vi "find greper points.vi"(2 "Circles":cluster{"x":dbl, "y":dbl, "r":dbl}[](array[cluster]), 3 "Type  2":enum16{"Z", "I", "O", "S", "L", "J", "T", "N"}(ring)=enum."O") -> (0 "gripper":T1, 1 "Type":enum16{"Z", "I", "O", "S", "L", "J", "T", "N"}(ring)=enum."O")   [LabVIEW 2018]
panel:
  out "output variable":i32
  out "dj":dbl[](array[numeric])
  out "di":dbl[](array[numeric])
  out "p2":dbl[](array[numeric])
  out "p1":dbl[](array[numeric])
  out "ok":i32
  out "i":i32
  out "points":cluster{"p1":dbl[], "p2":dbl[]}[](array[cluster])
  out "x":dbl[](array[numeric])
  out "y":dbl[](array[numeric])
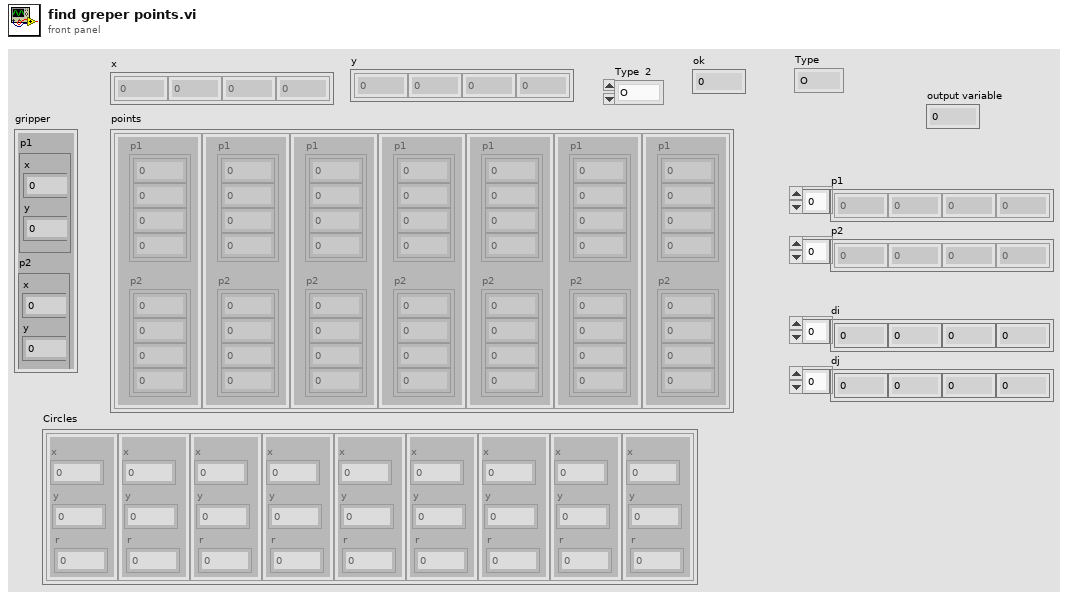
[diagram p1: front panel]
types:
  T1 = cluster{"p1":cluster{"x":dbl, "y":dbl}, "p2":cluster{"x":dbl, "y":dbl}}
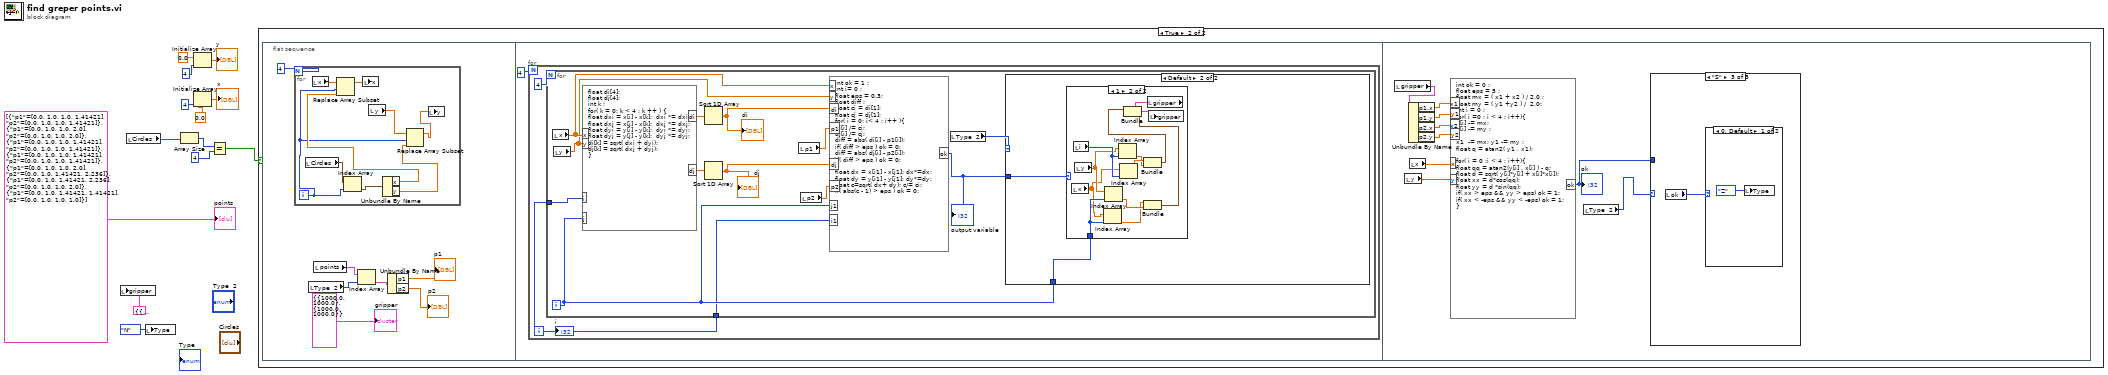
[diagram p0: block diagram]
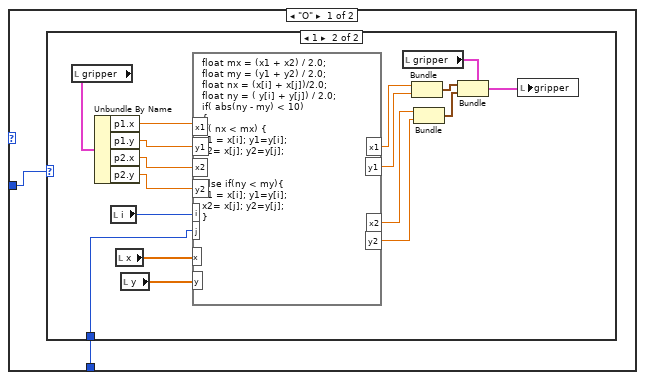
[diagram p3: hidden frame]
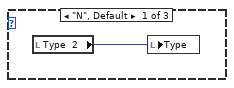
[diagram p6: hidden frame]
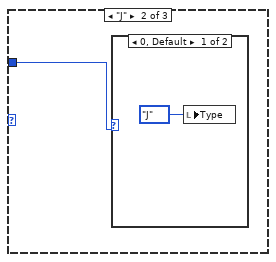
[diagram p7: hidden frame]
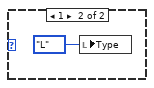
[diagram p8: hidden frame]
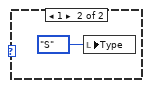
[diagram p9: hidden frame]
diagram:
  n1 = local write "gripper"(T1 {"p1"={"x"=0.0, "y"=0.0}, "p2"={"x"=0.0, "y"=0.0}} ("gripper")) -> ()
  n2 = local read "Circles"() -> (w13:cluster{"x":dbl, "y":dbl, "r":dbl}[])
  n3 = local write "Type"(enum16{"Z", "I", "O", "S", "L", "J", "T", "N"}."N" ("Type")) -> ()
  n4 = Array Size(array=w13) -> (size(s)=w12:i32)
  n5 = Initialize Array(0.0 ("element"), 4 ("dimension size")) -> (→"y":dbl[])
  n6 = Initialize Array(0.0 ("element"), 4 ("dimension size")) -> (→"x":dbl[])
  n7 = Equal?(x=w12, y=4) -> (x = y?=w10:bool)
  n8 = case shown="True" w10 {
    frame False {
    }
    frame True {
      n9 = flat-sequence {
        frame #0 {
          n10 = for {
            N: 4 -> [_]
            i -> [w23]
            n11 = local read "Circles"() -> (w29:cluster{"x":dbl, "y":dbl, "r":dbl}[])
            n12 = local read "x"() -> (w27:dbl[])
            n13 = Index Array(array=w29, index=w23) -> (element=w28:cluster{"x":dbl, "y":dbl, "r":dbl})
            n14 = local read "y"() -> (w24:dbl[])
            n15 = Unbundle By Name(w28) -> ("x"=w26:dbl, "y"=w22:dbl)
            n16 = Replace Array Subset(array=w27, new element=w26, index=w23) -> (w25:dbl[])
            n17 = local write "x"(w25) -> ()
            n18 = Replace Array Subset(array=w24, new element=w22, index=w23) -> (w21:dbl[])
            n19 = local write "y"(w21) -> ()
          }
          n20 = local read "Type  2"() -> (w18:enum16{"Z", "I", "O", "S", "L", "J", "T", "N"})
          n21 = local read "points"() -> (w19:cluster{"p1":dbl[], "p2":dbl[]}[])
          n22 = Index Array(array=w19, index=w18) -> (element=w17:cluster{"p1":dbl[], "p2":dbl[]})
          n23 = Unbundle By Name(w17) -> ("p1"=→"p1":dbl[], "p2"=→"p2":dbl[])
          "gripper" <- T1 {"p1"={"x"=1000.0, "y"=1000.0}, "p2"={"x"=1000.0, "y"=1000.0}} ("gripper")
        }
        frame #1 {
          n24 = for {
            N: 4 -> [_]
            i -> [w31]
            n25 = for {
              N: 4 -> [_]
              tunnel: w31 -> [w45]
              tunnel: w31 -> [w36]
              i -> [w37]
              n26 = local read "x"() -> (w35:dbl[])
              n27 = local read "y"() -> (w34:dbl[])
              n28 = formula code="float di[4];\nfloat dj[4];\nint k ;\nfor( k = 0; k < 4 ; k ++ ) {\nfloat dxi = x[i] - x[k];  dxi *= dxi;\nfloat dxj = x[j] - x[k];  dxj *= dxj;\nfloat dyi = y[i] - y[k];  dyi *= dyi;\nfloat dyj = y[j] - y[k];  dyj *= dyj;\ndi[k] = sqrt( dxi + dyi);\ndj[k] = sqrt( dxj + dyj);\n}"("i"=w45, "j"=w37, "x"=w35, "y"=w34) -> ("di"=w44:dbl[], "dj"=w43:dbl[])
              n29 = Sort 1D Array(array=w44) -> (sorted array=w42:dbl[])
              "di" <- w42
              n30 = Sort 1D Array(array=w43) -> (sorted array=w41:dbl[])
              "dj" <- w41
              n31 = local read "p1"() -> (w39:dbl[])
              n32 = local read "p2"() -> (w40:dbl[])
              n33 = formula code="int ok = 1 ;\nint i= 0 ;\nfloat eps = 0.3;\nfloat diff ;\nfloat ci = di[1];\nfloat cj = dj[1];\nfor( i = 0; i< 4 ; i++ ){\ndi[i] /= ci;\ndj[i] /= cj;\ndiff = abs( di[i] - p1[i]);\nif( diff > eps ) ok = 0;\ndiff = abs( dj[i] - p2[i]);\nif( diff > eps ) ok = 0;\n}\nfloat dx = x[i1] - x[j1]; dx*=dx;\nfloat dy = y[i1] - y[j1]; dy*=dy;\nfloat c=sqrt( dx+ dy); c/= ci;\nif( abs(c - 1) > eps ) ok = 0;"("di"=w42, "dj"=w41, "p1"=w39, "p2"=w40, "i1"=w36, "j1"=w37, "x"=w35, "y"=w34) -> ("ok"=w38:i32)
              "output variable" <- w38
              n34 = local read "Type  2"() -> (w33:enum16{"Z", "I", "O", "S", "L", "J", "T", "N"})
              n35 = case shown="Default" w33 {
                tunnel: w38 -> [w46 w66]
                tunnel: w37 -> [w47 w65]
                frame "O" {
                  n36 = case shown="1" w46 {
                    tunnel: w47 -> [_ w50]
                    frame 0, Default {
                    }
                    frame 1 {
                      n37 = local read "gripper"() -> (w60:T1)
                      n38 = Unbundle By Name(w60) -> ("p1.x"=w55:dbl, "p1.y"=w54:dbl, "p2.x"=w53:dbl, "p2.y"=w52:dbl)
                      n39 = local read "i"() -> (w51:i32)
                      n40 = local read "x"() -> (w49:dbl[])
                      n41 = local read "y"() -> (w48:dbl[])
                      n42 = formula code="float mx = (x1 + x2) / 2.0;\nfloat my = (y1 + y2) / 2.0;\nfloat nx = (x[i] + x[j])/2.0;\nfloat ny = ( y[i] + y[j]) / 2.0;\nif( abs(ny - my) < 10)\n{\nif( nx < mx) {\nx1 = x[i]; y1=y[i];\nx2= x[j]; y2=y[j];\n}\n}\nelse if(ny < my){\nx1 = x[i]; y1=y[i];\nx2= x[j]; y2=y[j];\n}"("x1"=w55, "y1"=w54, "x2"=w53, "y2"=w52, "i"=w51, "j"=w50, "x"=w49, "y"=w48) -> ("x1"=w59:dbl, "y1"=w58:dbl, "x2"=w57:dbl, "y2"=w56:dbl)
                      n43 = local read "gripper"() -> (w64:T1)
                      n44 = Bundle("x1"=w59, "y1"=w58) -> (w62:cluster{"x1":dbl, "y1":dbl})  [unwired: 1 in]
                      n45 = Bundle("x2"=w57, "y2"=w56) -> (w61:cluster{"x2":dbl, "y2":dbl})  [unwired: 1 in]
                      n46 = Bundle(cluster=w64, "p1"=w62, "p2"=w61) -> (w63:T1)
                      n47 = local write "gripper"(w63) -> ()
                    }
                  }
                }
                frame Default {
                  n48 = case shown="1" w66 {
                    tunnel: w65 -> [_ w76]
                    frame 0, Default {
                    }
                    frame 1 {
                      n49 = local read "x"() -> (w70:dbl[])
                      n50 = local read "i"() -> (w72:i32)
                      n51 = local read "y"() -> (w71:dbl[])
                      n52 = Index Array(array=w70, index=w76) -> (element=w73:dbl)
                      n53 = Index Array(array=w71, index=w76) -> (element=w74:dbl)
                      n54 = Index Array(array=w71, index=w72) -> (element=w68:dbl)
                      n55 = Index Array(array=w70, index=w72) -> (element=w69:dbl)
                      n56 = Bundle("element"=w69, "element"=w68) -> (w67:cluster{"element":dbl, "element":dbl})  [unwired: 1 in]
                      n57 = Bundle("element"=w73, "element"=w74) -> (w75:cluster{"element":dbl, "element":dbl})  [unwired: 1 in]
                      n58 = local read "gripper"() -> (w78:T1)
                      n59 = Bundle(cluster=w78, "p1"=w67, "p2"=w75) -> (w77:T1)
                      n60 = local write "gripper"(w77) -> ()
                    }
                  }
                }
              }
            }
            "i" <- w31
          }
        }
        frame #2 {
          n61 = local read "gripper"() -> (w87:T1)
          n62 = local read "y"() -> (w81:dbl[])
          n63 = Unbundle By Name(w87) -> ("p1.x"=w86:dbl, "p1.y"=w85:dbl, "p2.x"=w84:dbl, "p2.y"=w83:dbl)
          n64 = local read "x"() -> (w82:dbl[])
          n65 = formula code="int ok = 0 ;\nfloat eps = 5 ;\nfloat mx = ( x1 + x2 ) / 2.0 ;\nfloat my = ( y1 +y2 ) /  2.0;\nint i = 0 ;\nfor( i =0 ; i < 4 ; i++){\nx[i] -= mx;\ny[i] -= my ;\n}\nx1  -= mx; y1 -= my ;\nfloat q = atan2( y1 , x1);\n\nfor( i = 0 ;i < 4 ; i++){\nfloat qq = atan2(y[i] , x[i] ) - q;\nfloat d = sqrt( y[i]*y[i] + x[i]*x[i]);\nfloat xx = d*cos(qq);\nfloat yy = d *sin(qq);\nif( xx > eps && yy > eps) ok = 1;\nif( xx < -eps && yy < -eps) ok = 1;\n}"("x1"=w86, "y1"=w85, "x2"=w84, "y2"=w83, "x"=w82, "y"=w81) -> ("ok"=w79:i32)
          "ok" <- w79
          n66 = local read "Type  2"() -> (w80:enum16{"Z", "I", "O", "S", "L", "J", "T", "N"})
          n67 = case shown="\"S\"" w80 {
            tunnel: w79 -> [_ w89 _]
            frame "N", Default {
              n68 = local read "Type  2"() -> (w88:enum16{"Z", "I", "O", "S", "L", "J", "T", "N"})
              n69 = local write "Type"(w88) -> ()
            }
            frame "J" {
              n70 = case shown="0, Default" w89 {
                frame 0, Default {
                  n71 = local write "Type"(enum16{"Z", "I", "O", "S", "L", "J", "T", "N"}."J" ("Type  3")) -> ()
                }
                frame 1 {
                  n72 = local write "Type"(enum16{"Z", "I", "O", "S", "L", "J", "T", "N"}."L" ("Type  3")) -> ()
                }
              }
            }
            frame "S" {
              n73 = local read "ok"() -> (w92:i32)
              n74 = case shown="0, Default" w92 {
                frame 0, Default {
                  n75 = local write "Type"(enum16{"Z", "I", "O", "S", "L", "J", "T", "N"}."Z" ("Type  3")) -> ()
                }
                frame 1 {
                  n76 = local write "Type"(enum16{"Z", "I", "O", "S", "L", "J", "T", "N"}."S" ("Type  3")) -> ()
                }
              }
            }
          }
        }
      }
    }
  }
  "points" <- cluster{"p1":dbl[], "p2":dbl[]}[] [{"p1"=[0.0, 1.0, 1.0, 1.41421], "p2"=[0.0, 1.0, 1.0, 1.41421]}, {"p1"=[0.0, 1.0, 1.0, 2.0], "p2"=[0.0, 1.0, 1.0, 2.0]}, {"p1"=[0.0, 1.0, 1.0, 1.41421], "p2"=[0.0, 1.0, 1.0, 1.41421]}, {"p1"=[0.0, 1.0, 1.0, 1.41421], "p2"=[0.0, 1.0, 1.0, 1.41421]}, {"p1"=[0.0, 1.0, 1.0, 2.0], "p2"=[0.0, 1.0, 1.41421, 2.236]}, {"p1"=[0.0, 1.0, 1.41421, 2.236], "p2"=[0.0, 1.0, 1.0, 2.0]}, {"p1"=[0.0, 1.0, 1.41421, 1.41421], "p2"=[0.0, 1.0, 1.0, 1.0]}] ("points 2")
